vi "Fpga reg.vi"(8 "Mode":enum16{"Get", "Set"}(ring), 10 "FPGA VI Reference Set":T1) -> (2 "FPGA VI Reference Out":T1)   [LabVIEW 2019, in "my FPGA lib.lvlib"]
uses:
  my FPGA lib.lvlib
  FPPGA.ctl
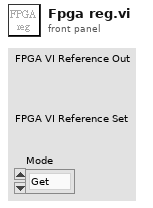
[diagram p1: front panel]
types:
  T1 = typedef "my FPGA lib.lvlib/FPPGA.ctl" = refnum<k20>
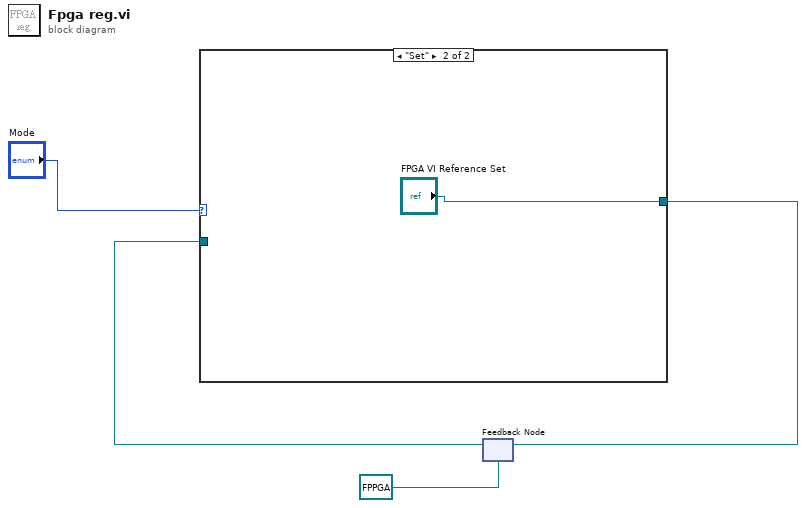
[diagram p0: block diagram]
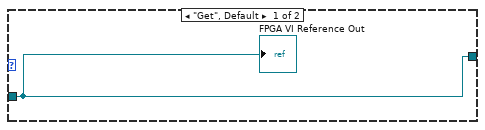
[diagram p2: hidden frame]
diagram:
  n1 = feedback #1(T1 refnum ("FPGA VI Reference Set")) -> (w2:T1)
  n2 = case shown="\"Set\"" "Mode" {
    tunnel: [w5 "FPGA VI Reference Set"] -> w3
    tunnel: w2 -> [w5 _]
    frame "Get", Default {
      "FPGA VI Reference Out" <- w5
    }
    frame "Set" {
    }
  }
  n3 = feedback-in #1(w3) -> ()
